vi "Destruct Messenger.vi"(8 "error in (no error)":errorcluster, 11 "Simple Map Queue Group Messenger Component in":refnum<class "Simple Map Queue Group Messenger.lvclass">) -> (0 "error out":errorcluster, 3 "Simple Map Queue Group Messenger Component out":refnum<class "Simple Map Queue Group Messenger.lvclass">)   [LabVIEW 2024, in "Simple Map Queue Group Messenger.lvclass"]
uses:
  Simple Map Queue Group Messenger.lvclass
  Simple Map Queue Group Messenger.lvclass/Simple Map Queue Group Messenger.ctl
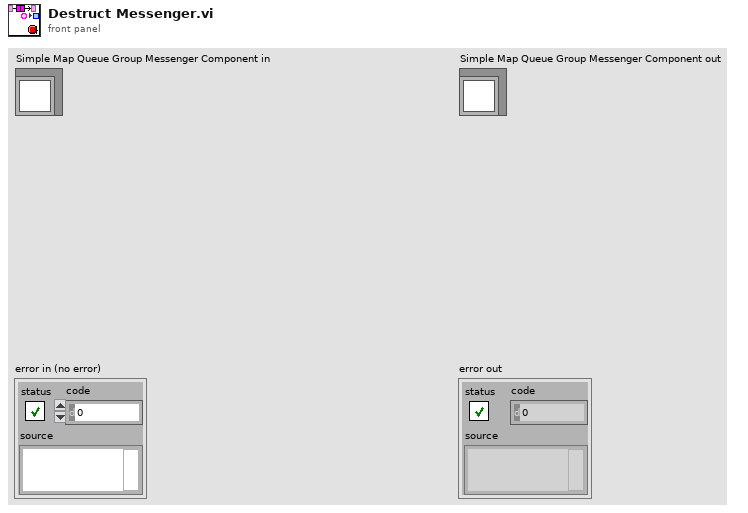
[diagram p1: front panel]
types:
  T1 = typedef "Queue Group Map.ctl" = map{i64, T2[]}
  T2 = typedef "Message Queue.ctl" = refnum<queue>
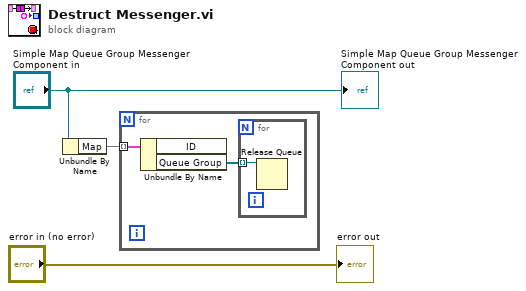
[diagram p0: block diagram]
diagram:
  n1 = Unbundle By Name("Simple Map Queue Group Messenger Component in") -> ("Map"=w1:T1)
  n2 = for {
    tunnel: w1 -> [w5] mode=indexing
    n3 = Unbundle By Name(w5) -> ("Queue Group"=w4:T2[])  [unwired: 1 out]
    n4 = for {
      tunnel: w4 -> [w6] mode=indexing
      n5 = Release Queue(queue=w6) -> ()  [unwired: 2 in, 3 out]
    }
  }
  "error out" <- "error in (no error)"
  "Simple Map Queue Group Messenger Component out" <- "Simple Map Queue Group Messenger Component in"
